vi "CheckPath.vi"(1 "Path":path) -> (0 "GoodPath":bool)   [LabVIEW 2013]
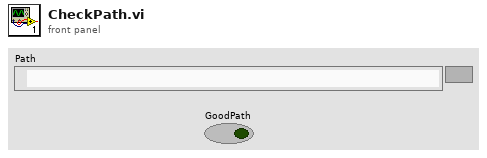
[diagram p1: front panel]
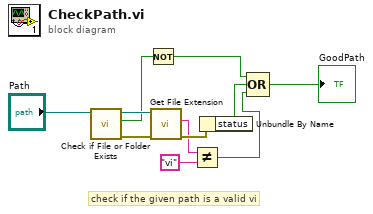
[diagram p0: block diagram]
diagram:
  # "check if the given path is a valid vi"
  n1 = call <vilib>:"Check if File or Folder Exists.vi"("path"="Path") -> ("error out"=w1:errorcluster, "file or folder exists?"=w4:bool, "dup path"=w11:path)  [unwired: 1 in, 7 out]
  n2 = Not(x=w4) -> (.not. x?=w7:bool)
  n3 = call <vilib>:"Get File Extension.vi"("error in (no error)"=w1, "file"=w11) -> ("error out"=w6:errorcluster, "lowercase file extension"=w3:string)  [unwired: 8 out]
  n4 = Not Equal?(x=w3, y="vi") -> (x != y?=w9:bool)
  n5 = Unbundle By Name(w6) -> ("status"=w8:bool)
  n6 = Compound Arithmetic op=OR(w7, w8, w9) -> (→"GoodPath":bool)
